vi "PixieGetHistograms.vi"(8 "error in (no error)":errorcluster, 10 "ModNum":u16) -> (0 "error out":errorcluster, 2 "Histogram Data":u32[][](array[numeric]))   [LabVIEW 2013]
uses:
  XIA/Pixie4/Drivers/Pixie4DLL.dll
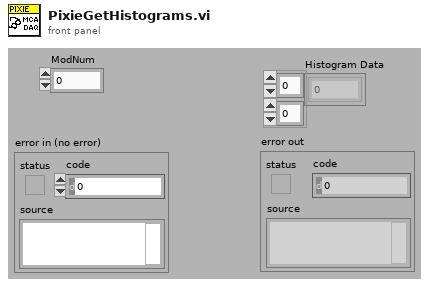
[diagram p1: front panel]
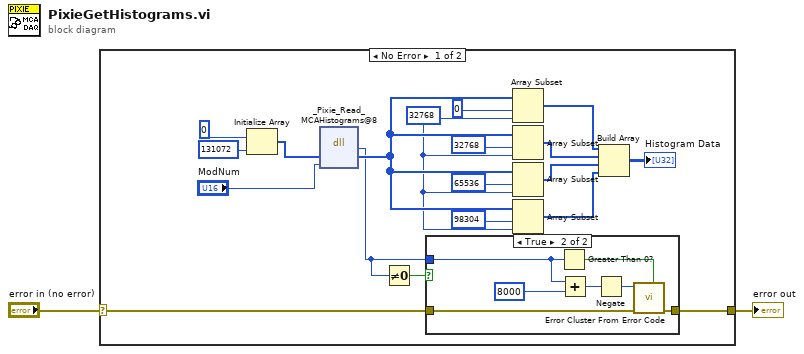
[diagram p0: block diagram]
diagram:
  n1 = case shown="No Error" "error in (no error)" {
    selector: "error in (no error)" -> [w4 w30]
    tunnel: [w5 w30] -> w1
    frame No Error {
      w17 = 32768
      n2 = Initialize Array(u32 0, 131072) -> (w7:u32[])
      n3 = dll-call lib="C:/XIA/Pixie4/Drivers/Pixie4DLL.dll" fn="_Pixie_Read_MCAHistograms@8"("MCAHistograms"=w7, "ModNum"="ModNum") -> ("return type"=w3:i32, "MCAHistograms"=w18:u32[])  [unwired: 4 in, 2 out]
      n4 = Not Equal To 0?(x=w3) -> (x != 0?=w6:bool)
      n5 = case shown="True" w6 {
        tunnel: [w22 w25] -> w5
        tunnel: w4 -> [w22 w24]
        tunnel: w3 -> [_ w23]
        frame False {
        }
        frame True {
          n6 = Greater Than 0?(x=w23) -> (x > 0?=w27:bool)
          n7 = Add(x=w23, y=8000) -> (x+y=w28:i32)
          n8 = Negate(x=w28) -> (-x=w26:i32)
          n9 = call <vilib>:"Error Cluster From Error Code.vi"("is warning? (False)"=w27, "error in (no error)"=w24, "error code (0)"=w26) -> ("error out"=w25:errorcluster)  [unwired: 1 in, 5 out]
        }
      }
      n10 = Array Subset(array=w18, index=0, length=w17) -> (w12:u32[])
      n11 = Array Subset(array=w18, index=32768, length=w17) -> (w11:u32[])
      n12 = Array Subset(array=w18, index=65536, length=w17) -> (w10:u32[])
      n13 = Array Subset(array=w18, index=98304, length=w17) -> (w9:u32[])
      n14 = Build Array(w12, w11, w10, w9) -> (→"Histogram Data":u32[][])
    }
    frame Error {
    }
  }
  "error out" <- w1
